vi "FPGA UTF 8 Test.vi"() -> ()   [LabVIEW 2022 SP3]
panel:
  out "Pwr ±15V Primary Err":bool
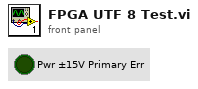
[diagram p1: front panel]
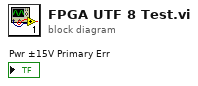
[diagram p0: block diagram]
diagram:
